vi "RemovePoint.vi"(8 "Amp in":dbl[](array[numeric]), 9 "Y in":u32[](array[numeric]), 10 "X in":u32[](array[numeric]), 11 "Index":i32) -> (0 "Amp out":dbl[](array[numeric]), 1 "Y out":u32[](array[numeric]), 2 "X out":u32[](array[numeric]))   [LabVIEW 2017, in "AODControl.lvlib"]
uses:
  AODControl.lvlib
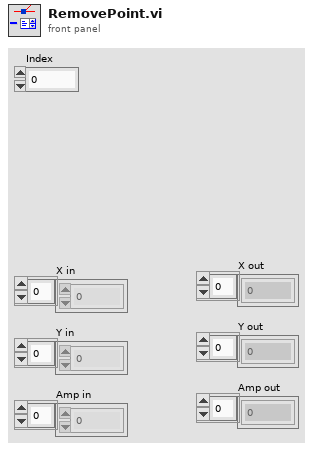
[diagram p1: front panel]
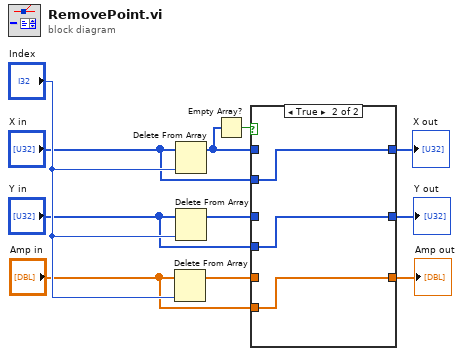
[diagram p0: block diagram]
diagram:
  n1 = Delete From Array(array="Amp in", index="Index") -> (array with subset deleted=w4:dbl[])  [unwired: 1 in, 1 out]
  n2 = Delete From Array(array="X in", index="Index") -> (array with subset deleted=w6:u32[])  [unwired: 1 in, 1 out]
  n3 = Delete From Array(array="Y in", index="Index") -> (array with subset deleted=w5:u32[])  [unwired: 1 in, 1 out]
  n4 = Empty Array?(array=w6) -> (empty?=w7:bool)
  n5 = case shown="True" w7 {
    tunnel: w6 -> [w14 _]
    tunnel: [w14 w17] -> w10
    tunnel: [w13 w16] -> w9
    tunnel: w5 -> [w13 _]
    tunnel: [w12 w15] -> w8
    tunnel: w4 -> [w12 _]
    tunnel: "X in" -> [_ w17]
    tunnel: "Y in" -> [_ w16]
    tunnel: "Amp in" -> [_ w15]
    frame False {
    }
    frame True {
    }
  }
  "Amp out" <- w8
  "Y out" <- w9
  "X out" <- w10
